vi "_OBSOLETE_PathPlanner_Trajectory_CalculateVelocity.vi"(9 "MaxAccel":dbl, 10 "PathPoints":T1[](array[typedef]) {"HolonomicRotation"."SIN" format="%13.4f"; "HolonomicRotation"."COS" format="%13.4f"; "HolonomicRotation"."VALUE" format="%13.4f"; "NextControl"."Y" format="%14.3f"; "NextControl"."X" format="%14.3f"; "PrevControl"."Y" format="%14.3f"; "PrevControl"."X" format="%14.3f"; "AnchorPoint"."Y" format="%14.3f"; "AnchorPoint"."X" format="%14.3f"}, 11 "PathPlannerStates":T4[](array[typedef]) {"TargetHolonomicRotation"."SIN" format="%13.4f"; "TargetHolonomicRotation"."COS" format="%13.4f"; "TargetHolonomicRotation"."VALUE" format="%13.4f"; "Heading"."SIN" format="%13.4f"; "Heading"."COS" format="%13.4f"; "Heading"."VALUE" format="%13.4f"; "PositionMeters"."Y" format="%14.3f"; "PositionMeters"."X" format="%14.3f"}) -> (3 "outPathPlannerStates":T4[](array[typedef]) {"TargetHolonomicRotation"."SIN" format="%13.4f"; "TargetHolonomicRotation"."COS" format="%13.4f"; "TargetHolonomicRotation"."VALUE" format="%13.4f"; "Heading"."SIN" format="%13.4f"; "Heading"."COS" format="%13.4f"; "Heading"."VALUE" format="%13.4f"; "PositionMeters"."Y" format="%14.3f"; "PositionMeters"."X" format="%14.3f"})   [LabVIEW 2019]
uses:
  <vilib>/Rock Robotics/WPI/ThirdParty/JAS_Junk/TrajLib/TypeDef/ROTATION2D.ctl
  <vilib>/Rock Robotics/WPI/ThirdParty/JAS_Junk/TrajLib/Trajectory_Library.lvlib
  <vilib>/Rock Robotics/WPI/ThirdParty/JAS_Junk/TrajLib/TypeDef/TRANSLATION2D.ctl
  TypeDef/PathPlannerTrajectoryState.ctl
  PathPlanner24.lvlib
  TypeDef/PathPlannerWaypoint.ctl
  TypeDef/PathPlannerPathConstraints.ctl
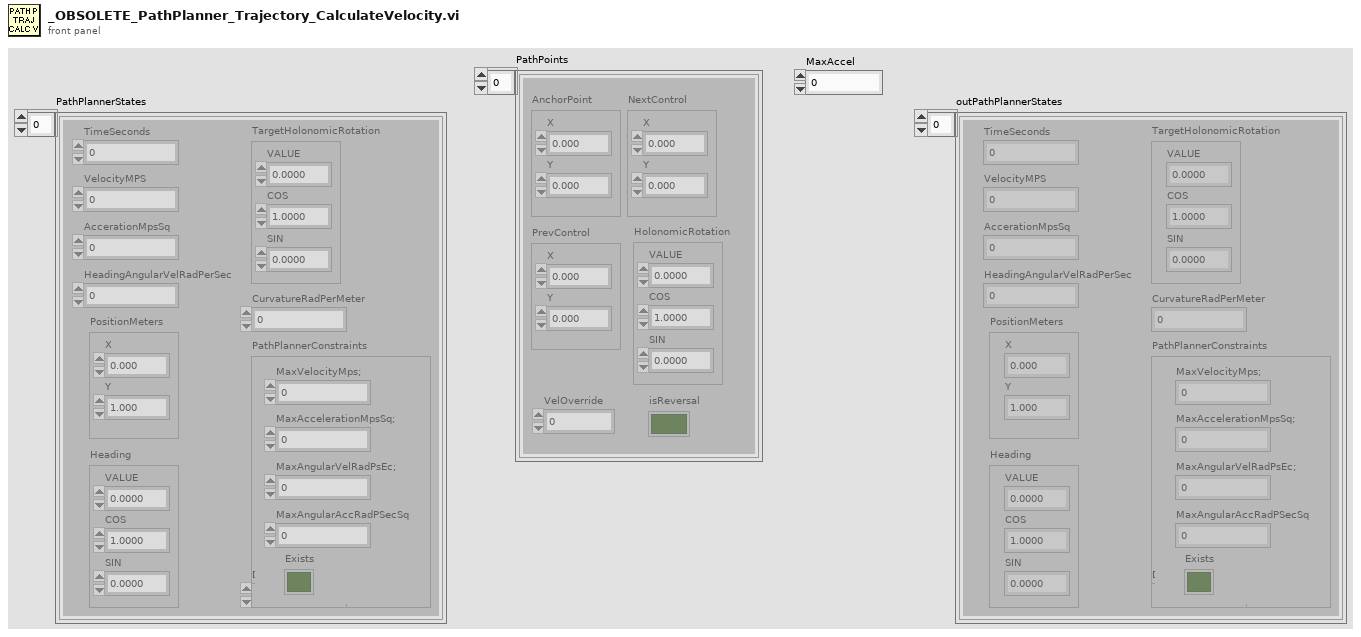
[diagram p1: front panel]
types:
  T1 = typedef "PathPlanner24.lvlib/PathPlannerWaypoint.ctl" = cluster{"AnchorPoint":T2, "PrevControl":T2, "NextControl":T2, "HolonomicRotation":T3, "VelOverride":dbl, "isReversal":bool}
  T2 = typedef "Trajectory_Library.lvlib/TRANSLATION2D.ctl" = cluster{"X":dbl, "Y":dbl}
  T3 = typedef "Trajectory_Library.lvlib/ROTATION2D.ctl" = cluster{"VALUE":dbl, "COS":dbl, "SIN":dbl}
  T4 = typedef "PathPlanner24.lvlib/PathPlannerTrajectoryState.ctl" = cluster{"TimeSeconds":dbl, "VelocityMPS":dbl, "AccerationMpsSq":dbl, "HeadingAngularVelRadPerSec":dbl, "PositionMeters":T2, "Heading":T3, "TargetHolonomicRotation":T3, "CurvatureRadPerMeter":dbl, "DeltaPos":dbl, "PathPlannerConstraints":T5}
  T5 = typedef "PathPlanner24.lvlib/PathPlannerPathConstraints.ctl" = cluster{"MaxVelocityMps;":dbl, "MaxAccelerationMpsSq;":dbl, "MaxAngularVelRadPsEc;":dbl, "MaxAngularAccRadPSecSq":dbl, "Exists":bool}
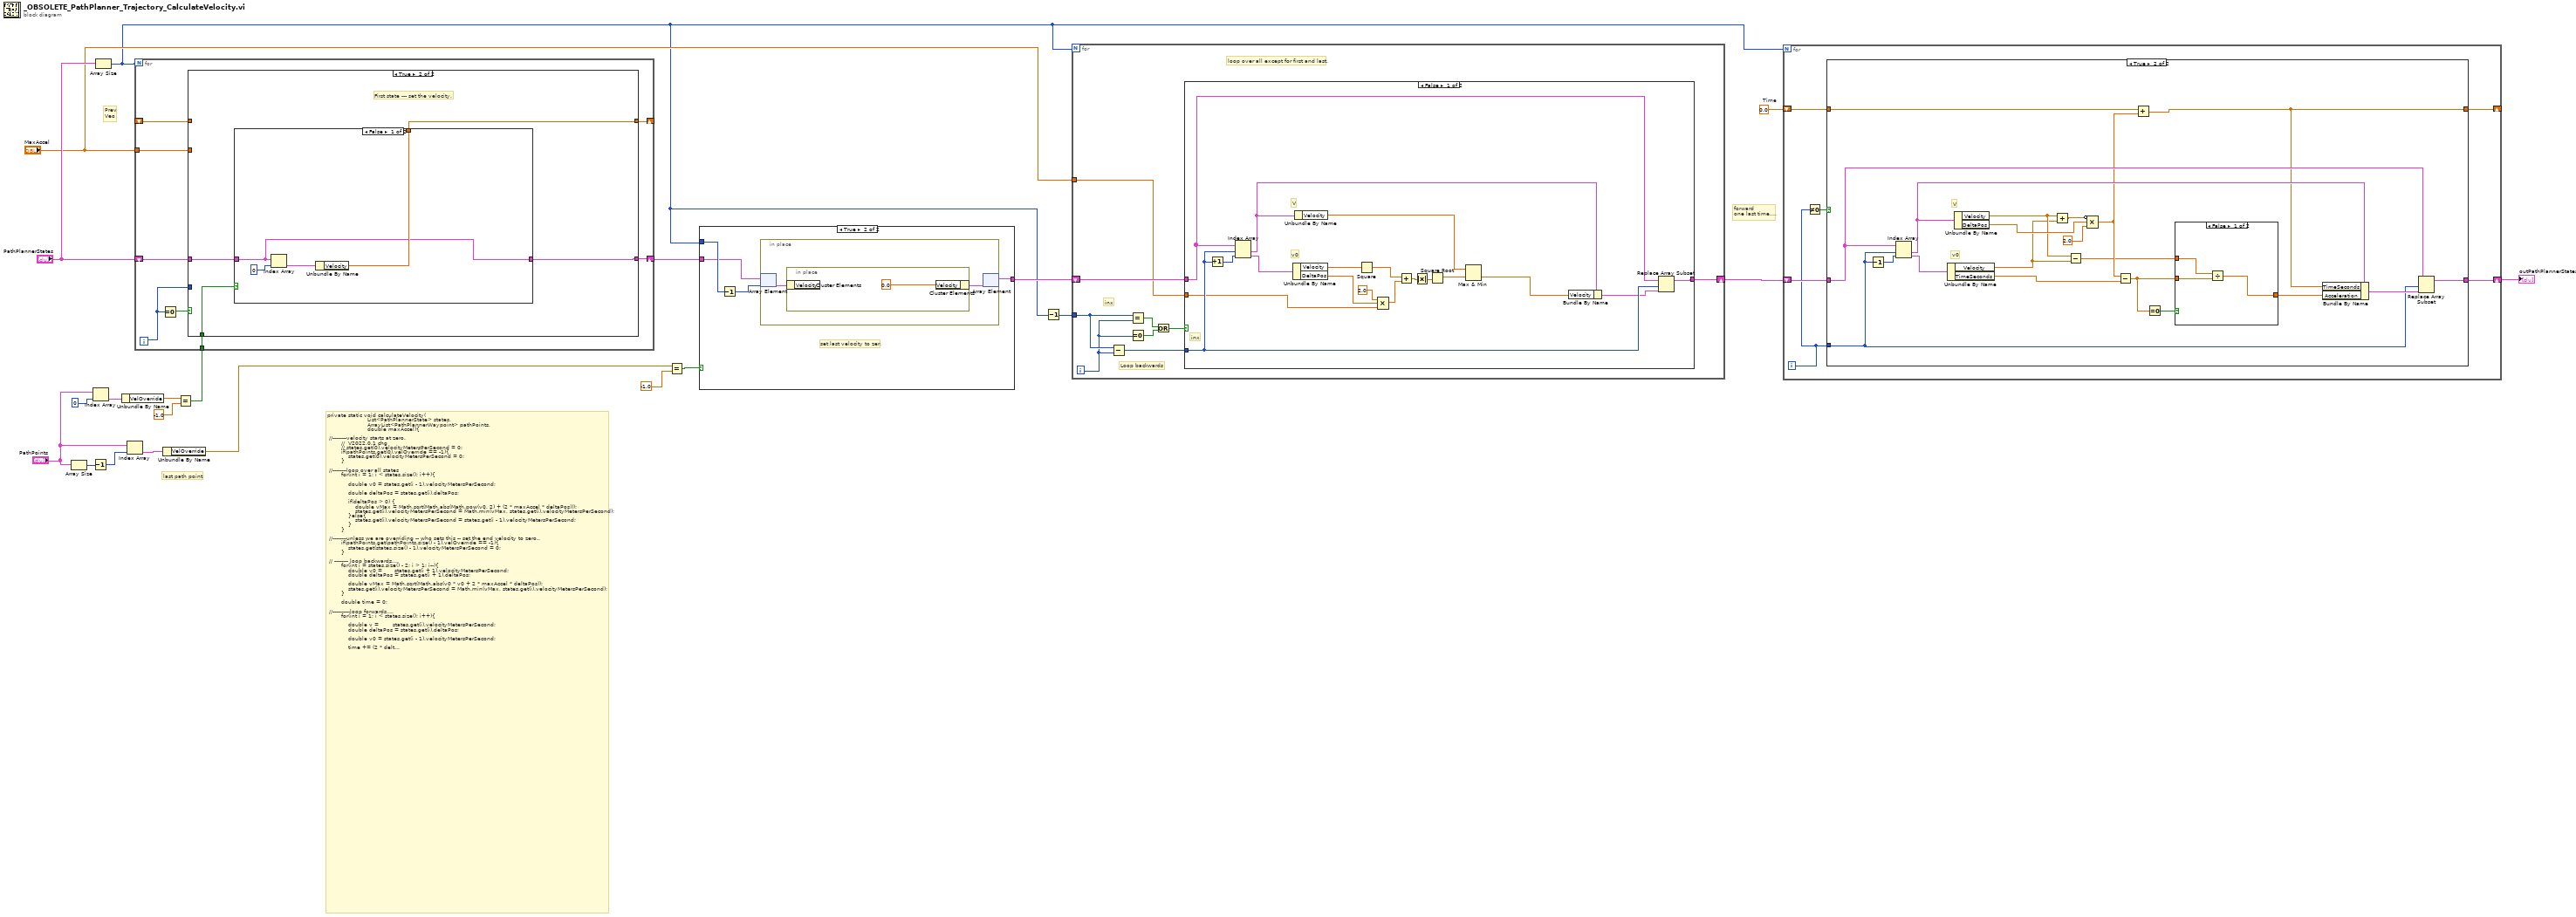
[diagram p0: block diagram]
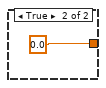
[diagram p3: hidden frame]
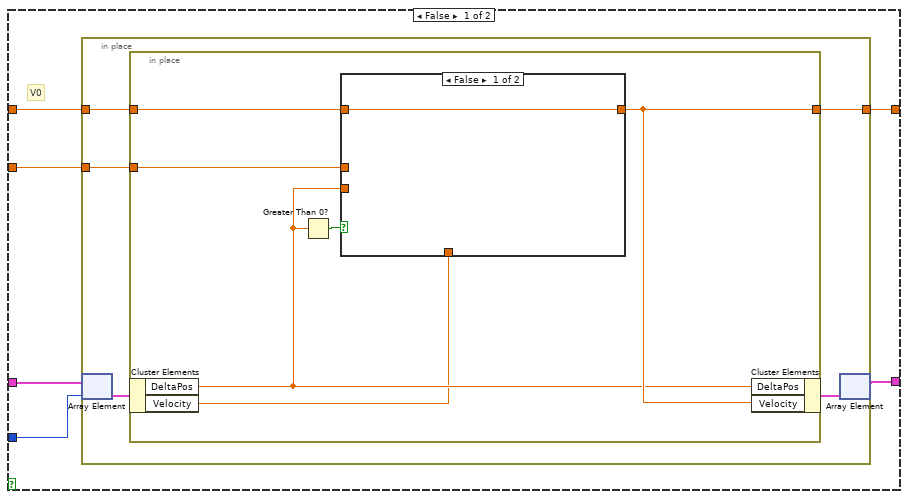
[diagram p6: hidden frame]
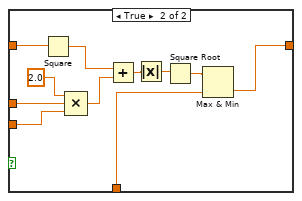
[diagram p7: hidden frame]
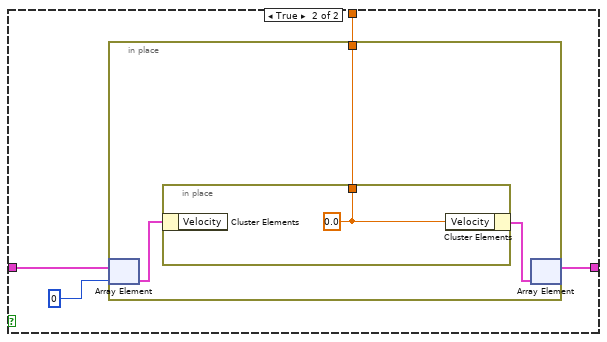
[diagram p8: hidden frame]
diagram:
  w10 = 0.0  # Time
  # "last path point"
  # "private static void calculateVelocity(\n\t\t                     List<PathPlannerState> states, \n\t\t                     ArrayList<PathPlannerWaypoint> pathPoints, \n\t\t                     double maxAccel){\n\n\t//--------velocity starts at zero.\n        //  V2022.0.1 chg\n        // states.get(0).velocityMetersPerSecond = 0;\n        if(pathPoints.get(0).velOverride == -1){\n            states.get(0).velocityMetersPerSecond = 0;\n        }\n\n\t//--------loop over all states\n        for(int i = 1; i < states.size(); i++){\n\n            double v0 = states.get(i - 1).velocityMetersPerSecond;\n\n            double deltaPos = states.get(i).deltaPos;\n\n            if(deltaPos > 0) {\n                double vMax = Math.sqrt(Math.abs(Math.pow(v0, 2) + (2 * maxAccel * deltaPos)));\n                states.get(i).velocityMetersPerSecond = Math.min(vMax, states.get(i).velocityMetersPerSecond);\n            }else{\n                states.get(i).velocityMetersPerSecond = states.get(i - 1).velocityMetersPerSecond;\n            }\n        }\n\n\t//--------unless we are overriding -- who sets this -- set the end velocity to zero..\n        if(pathPoints.get(pathPoints.size() - 1).velOverride == -1){\n            states.get(states.size() - 1).velocityMetersPerSecond = 0;\n        }\n\n\t// -------- loop backwards....\n        for(int i = states.size() - 2; i > 1; i--){\n            double v0 =       states.get(i + 1).velocityMetersPerSecond;\n            double deltaPos = states.get(i + 1).deltaPos;\n\n            double vMax = Math.sqrt(Math.abs(v0 * v0 + 2 * maxAccel * deltaPos));\n            states.get(i).velocityMetersPerSecond = Math.min(vMax, states.get(i).velocityMetersPerSecond);\n        }\n\n        double time = 0;\n\n\t//----------loop forwards....\n        for(int i = 1; i < states.size(); i++){\n\n            double v =        states.get(i).velocityMetersPerSecond;\n            double deltaPos = states.get(i).deltaPos;\n\n            double v0 = states.get(i - 1).velocityMetersPerSecond;\n\n            time += (2 * deltaPos) / (v + v0);\n\n            states.get(i).timeSeconds = time;\n\n            double dv = v - v0;\n            double dt = time - states.get(i - 1).timeSeconds;\n\n            if(dt == 0){\n                states.get(i).accelerationMetersPerSecondSq = 0;\n            }else{\n                states.get(i).accelerationMetersPerSecondSq = dv / dt;\n            }\n        }\n    }"
  # "forward\none last time...."
  # "Prev\nVeo"
  n1 = Array Size(array="PathPoints") -> (size(s)=w20:i32)
  n2 = Index Array(array="PathPoints", index=0) -> (element=w4:T1)
  n3 = Decrement(x=w20) -> (x-1=w19:i32)
  n4 = Array Size(array="PathPlannerStates") -> (size(s)=w7:i32)
  n5 = Unbundle By Name(w4) -> ("VelOverride"=w3:dbl)
  n6 = Index Array(array="PathPoints", index=w19) -> (element=w18:T1)
  n7 = Unbundle By Name(w18) -> ("VelOverride"=w15:dbl)
  n8 = Equal?(x=w3, y=-1.0) -> (x = y?=w1:bool)
  n9 = for {
    N: w7 -> [_]
    shift-right: [w27] -> w14
    shift-left: "PathPlannerStates" -> [w28]
    shift-right: [w26] -> _
    shift-left: _ -> [w24]
    tunnel: "MaxAccel" -> [w23]
    tunnel: w1 -> [w22]
    i -> [w25]
    n10 = Equal To 0?(x=w25) -> (x = 0?=w29:bool)
    n11 = case shown="True" w29 {
      tunnel: w28 -> [w32 w62]
      tunnel: [w30 w61] -> w27
      tunnel: [w34 w60] -> w26
      tunnel: w25 -> [w31 _]
      tunnel: w24 -> [w35 _]
      tunnel: w23 -> [w33 _]
      tunnel: w22 -> [_ w59]
      frame False {
        # "V0"
        n12 = in-place {
          in-place-border: w35 -> [w40]
          in-place-border: [w39] -> w34
          in-place-border: w33 -> [w38]
          n13 = in-place-array #1(w32, w31) -> (w37:T4)
          n14 = in-place {
            in-place-border: w40 -> [w45]
            in-place-border: [w44] -> w39
            in-place-border: w38 -> [w43]
            n15 = in-place-cluster #2(w37) -> ("DeltaPos"=w42:dbl, "Velocity"=w41:dbl)
            n16 = Greater Than 0?(x=w42) -> (x > 0?=w46:bool)
            n17 = case shown="False" w46 {
              tunnel: w45 -> [w47 w58]
              tunnel: [w47 w50] -> w44
              tunnel: w43 -> [_ w56]
              tunnel: w42 -> [_ w55]
              tunnel: w41 -> [_ w51]
              frame False {
              }
              frame True {
                n18 = Square(x=w58) -> (x^2=w54:dbl)
                n19 = Compound Arithmetic op=MULTIPLY(2.0 ("value"), w56, w55) -> (w53:dbl)
                n20 = Add(x=w54, y=w53) -> (x+y=w48:dbl)
                n21 = Absolute Value(x=w48) -> (abs(x)=w49:dbl)
                n22 = Square Root(x=w49) -> (sqrt(x)=w52:dbl)
                n23 = Max & Min(x=w52, y=w51) -> (min(x,y)=w50:dbl)  [unwired: 1 out]
              }
            }
            n24 = in-place-cluster #2("DeltaPos"=w42, "Velocity"=w44) -> (w36:T4)
          }
          n25 = in-place-array #1(w36) -> (w30:T4[])  [unwired: 1 out]
        }
      }
      frame True {
        # "First state --- set the velocity."
        n26 = case shown="False" w59 {
          tunnel: w62 -> [w63 w70]
          tunnel: [w63 w69] -> w61
          tunnel: [w64 w67] -> w60
          frame False {
            n27 = Index Array(array=w63, index=0) -> (element=w65:T4)
            n28 = Unbundle By Name(w65) -> ("Velocity"=w64:dbl)
          }
          frame True {
            n29 = in-place {
              in-place-border: [w72] -> w67
              n30 = in-place-array #3(w70, 0) -> (w71:T4)
              n31 = in-place {
                in-place-border: [w74] -> w72
                w74 = 0.0 ("TrajectoryState.Velocity")
                n32 = in-place-cluster #4(w71) -> ()  [unwired: 1 out]
                n33 = in-place-cluster #4("Velocity"=w74) -> (w73:T4)
              }
              n34 = in-place-array #3(w73) -> (w69:T4[])  [unwired: 1 out]
            }
          }
        }
      }
    }
  }
  n35 = Equal?(x=w15, y=-1.0) -> (x = y?=w17:bool)
  n36 = case shown="True" w17 {
    tunnel: w14 -> [w75 w78]
    tunnel: w7 -> [_ w79]
    tunnel: [w75 w77] -> w13
    frame False {
    }
    frame True {
      # "set last velocity to zer."
      n37 = Decrement(x=w79) -> (x-1=w76:i32)
      n38 = in-place {
        n39 = in-place-array #5(w78, w76) -> (w81:T4)
        n40 = in-place {
          n41 = in-place-cluster #6(w81) -> ()  [unwired: 1 out]
          n42 = in-place-cluster #6("Velocity"=0.0 ("TrajectoryState.Velocity")) -> (w80:T4)
        }
        n43 = in-place-array #5(w80) -> (w77:T4[])  [unwired: 1 out]
      }
    }
  }
  n44 = Decrement(x=w7) -> (x-1=w12:i32)
  n45 = for {
    N: w7 -> [_]
    shift-right: [w85] -> w11
    shift-left: w13 -> [w86]
    tunnel: w12 -> [w91]
    tunnel: "MaxAccel" -> [w84]
    i -> [w83]
    # "loop over all except for first and last."
    # "inx"
    # "Loop backwards"
    n46 = Subtract(x=w91, y=w83) -> (x-y=w87:i32)
    n47 = Equal?(x=w91, y=w83) -> (x = y?=w90:bool)
    n48 = Equal To 0?(x=w83) -> (x = 0?=w89:bool)
    n49 = Or(x=w90, y=w89) -> (x .or. y?=w88:bool)
    n50 = case shown="False" w88 {
      tunnel: w87 -> [w104 _]
      tunnel: w86 -> [w105 w110]
      tunnel: [w107 w110] -> w85
      tunnel: w84 -> [w99 _]
      frame False {
        # "v0"
        # "V"
        # "inx"
        n51 = Increment(x=w104) -> (x+1=w109:i32)
        n52 = Index Array(array=w105, index #1=w104, index #2=w109) -> (element #1=w106:T4, element #2=w108:T4)
        n53 = Unbundle By Name(w108) -> ("Velocity"=w102:dbl, "DeltaPos"=w100:dbl)
        n54 = Unbundle By Name(w106) -> ("Velocity"=w94:dbl)
        n55 = Square(x=w102) -> (x^2=w98:dbl)
        n56 = Compound Arithmetic op=MULTIPLY(2.0 ("value"), w100, w99) -> (w97:dbl)
        n57 = Add(x=w98, y=w97) -> (x+y=w93:dbl)
        n58 = Absolute Value(x=w93) -> (abs(x)=w92:dbl)
        n59 = Square Root(x=w92) -> (sqrt(x)=w96:dbl)
        n60 = Max & Min(x=w94, y=w96) -> (min(x,y)=w95:dbl)  [unwired: 1 out]
        n61 = Bundle By Name(cluster=w106, "Velocity"=w95) -> (w103:T4)
        n62 = Replace Array Subset(array=w105, new element=w103, index=w104) -> (w107:T4[])
      }
      frame True {
        # "For first and last states, do nothing."
      }
    }
  }
  n63 = for {
    N: w7 -> [_]
    shift-right: [w115] -> w8
    shift-left: w11 -> [w116]
    shift-right: [w113] -> _
    shift-left: w10 -> [w114]
    i -> [w111]
    n64 = Not Equal To 0?(x=w111) -> (x != 0?=w112:bool)
    n65 = case shown="True" w112 {
      tunnel: w116 -> [w117 w138]
      tunnel: [w117 w137] -> w115
      tunnel: w114 -> [w118 w129]
      tunnel: [w118 w119] -> w113
      tunnel: w111 -> [_ w120]
      frame False {
        # "first time.... do nothing..."
      }
      frame True {
        # "v0"
        # "V"
        n66 = Decrement(x=w120) -> (x-1=w136:i32)
        n67 = Index Array(array=w138, index #1=w120, index #2=w136) -> (element #1=w134:T4, element #2=w135:T4)
        n68 = Unbundle By Name(w135) -> ("Velocity"=w127:dbl, "TimeSeconds"=w126:dbl)
        n69 = Unbundle By Name(w134) -> ("Velocity"=w128:dbl, "DeltaPos"=w131:dbl)
        n70 = Add(x=w128, y=w127) -> (x+y=w132:dbl)
        n71 = Subtract(x=w128, y=w127) -> (x-y=w122:dbl)
        n72 = Compound Arithmetic op=MULTIPLY(invert w132, w131, 2.0 ("value")) -> (w125:dbl)
        n73 = Subtract(x=w125, y=w126) -> (x-y=w121:dbl)
        n74 = Add(x=w129, y=w125) -> (x+y=w119:dbl)
        n75 = Equal To 0?(x=w121) -> (x = 0?=w124:bool)
        n76 = case shown="False" w124 {
          tunnel: [w139 0.0] -> w123
          tunnel: w122 -> [w141 _]
          tunnel: w121 -> [w140 _]
          frame False {
            n77 = Divide(x=w141, y=w140) -> (x/y=w139:dbl)
          }
          frame True {
          }
        }
        n78 = Bundle By Name(cluster=w134, "TimeSeconds"=w119, "Acceleration"=w123) -> (w133:T4)
        n79 = Replace Array Subset(array=w138, new element=w133, index=w120) -> (w137:T4[])
      }
    }
  }
  "outPathPlannerStates" <- w8
